vi "DH_Forward Kinematics.vi"(0 "start pose":T1=[[1.0, 0.0, 0.0, 0.0], [0.0, 1.0, 0.0, 0.0], [0.0, 0.0, 1.0, 0.0], [0.0, 0.0, 0.0, 1.0]], 2 "Joints":T2(array[cluster])) -> (4 "Intermediate Poses":dbl[][][](array[numeric]), 5 "end effector pose":T1=[[0.2818556107229001, -0.49341675968208987, -0.8228592321708784, 0.11697004227643469], [-0.7778734424176673, -0.6195744782940995, 0.10507318129704712, 0.030499600323496263], [-0.5616674481268332, 0.6104648778688426, -0.5584463363683838, -0.2863453905069739], [0.0, 0.0, 0.0, 1.0]] format="%#_2g", 6 "z_i":dbl[][](array[numeric]), 7 "positions":dbl[][](array[numeric]))   [LabVIEW 2024]
uses:
  <vilib>/Analysis/Matrix/Datatypes/RealMatrix.ctl
  <vilib>/Analysis/Matrix/NI_Matrix.lvlib
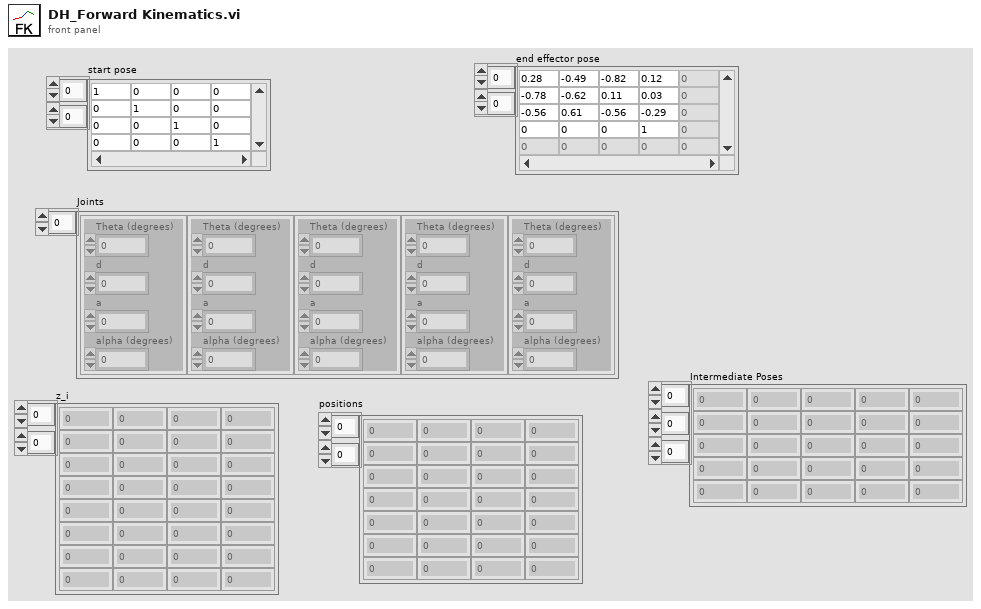
[diagram p1: front panel]
types:
  T1 = typedef "NI_Matrix.lvlib/RealMatrix.ctl" = dbl[][]
  T2 = cluster{"Theta (degrees)":dbl, "d":dbl, "a":dbl, "alpha (degrees)":dbl}[]
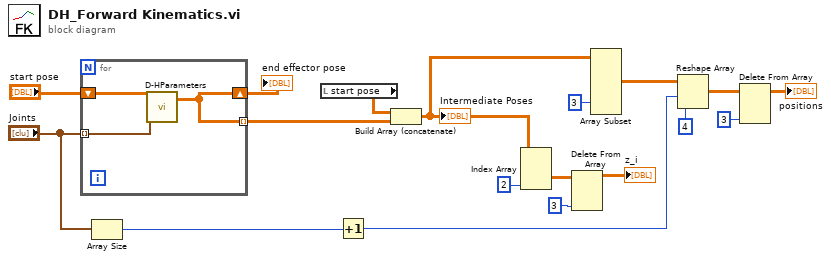
[diagram p0: block diagram]
diagram:
  n1 = for {
    shift-right: [w19] -> w18
    shift-left: "start pose" -> [w20]
    tunnel: "Joints" -> [w21] mode=indexing
    tunnel: [w19] -> w17 mode=indexing
    n2 = call <userlib>:"D-HParameters.vi"("n+1"=w21, "Start"=w20) -> ("A x B"=w19:T1)  [unwired: 1 out]
  }
  "end effector pose" <- w18
  n3 = Array Size(array="Joints") -> (size(s)=w10:i32)
  n4 = local read "start pose"() -> (w15:T1)
  n5 = Increment(x=w10) -> (x+1=w2:i32)
  n6 = Build Array (concatenate)(w15, w17) -> (w1:dbl[][][])
  "Intermediate Poses" <- w1
  n7 = Index Array(array=w1, index (dim 2)=2 ("disabled index (col)")) -> (element=w4:dbl[][])  [unwired: 2 in]
  n8 = Delete From Array(array=w4, index (col)=3 ("disabled index (col)")) -> (array with subset deleted=→"z_i":dbl[][])  [unwired: 2 in, 1 out]
  n9 = Array Subset(array=w1, index (dim 2)=3 ("index")) -> (w12:dbl[][][])  [unwired: 5 in]
  n10 = Reshape Array(w12, w2, 4 ("index")) -> (w8:dbl[][])
  n11 = Delete From Array(array=w8, index (col)=3 ("disabled index (col)")) -> (array with subset deleted=→"positions":dbl[][])  [unwired: 2 in, 1 out]
